vi "ReadAddErrorCase__slk_mt.vi"(8 "error in (no error)":errorcluster, 11 "refnum in":T1) -> (0 "error out":errorcluster, 2 "add error case configure":T2, 3 "refnum out":T1)   [LabVIEW 2020, in "Lazyboots Menu Tool.lvlib"]
doc: "Gets configure datum of Add Error Case.\n\n<b>[Add Error Case]</b>\nFrame Width = \"20\"\nCreate Constant = \"TRUE\""
uses:
  Library/Lazyboots Menu Tool.lvlib
  TypeDef/TypeDef_AddErrorCaseConfigure__slk_mt.ctl
  <vilib>/Utility/config.llb/Config Data RefNum.ctl
  <vilib>/Utility/config.llb/Read Key (U32).vi
  <vilib>/Utility/config.llb/Read Key (Boolean).vi
  <vilib>/Utility/config.llb/NI_LVConfig.lvlib
panel:
  # "ReadAddErrorCase__slk_mt.vi\nGets configure datum of Add Error Case.\n\nNOTICE -- YOU MUST LEAVE THIS NOTICE IN PLACE.\n\nCopyright (c) 2011, LIANG LIU Shawn.Liu.cn@gmail.com\nAll rights reserved.\n\nRedistribution and use in source and binary forms, with or without modification, are permitted provided that the following conditions are met:\n-Redistributions of source code must retain the above copyright notice, this list of conditions and the following disclaimer.\n-Redistributions in binary form must reproduce the above copyright notice, this list of conditions and the following disclaimer in the documentation and/or other materials provided with the distribution.\n-Neither the name of the eLp nor the names of its contributors may be used to endorse or promote products derived from this software without specific prior written permission.\n\nTHIS SOFTWARE IS PROVIDED BY THE COPYRIGHT HOLDERS AND CONTRIBUTORS \"AS IS\" AND ANY EXPRESS OR IMPLIED WARRANTIES, INCLUDING, BUT NOT LIMITED TO, THE IMPLIED WARRANTIES OF MERCHANTABILITY AND FITNESS FOR A PARTICULAR PURPOSE ARE DISCLAIMED. IN NO EVENT SHALL THE COPYRIGHT HOLDER OR CONTRIBUTORS BE LIABLE FOR ANY DIRECT, INDIRECT, INCIDENTAL, SPECIAL, EXEMPLARY, OR CONSEQUENTIAL DAMAGES (INCLUDING, BUT NOT LIMITED TO, PROCUREMENT OF SUBSTITUTE GOODS OR SERVICES; LOSS OF USE, DATA, OR PROFITS; OR BUSINESS INTERRUPTION) HOWEVER CAUSED AND ON ANY THEORY OF LIABILITY, WHETHER IN CONTRACT, STRICT LIABILITY, OR TORT (INCLUDING NEGLIGENCE OR OTHERWISE) ARISING IN ANY WAY OUT OF THE USE OF THIS SOFTWARE, EVEN IF ADVISED OF THE POSSIBILITY OF SUCH DAMAGE."
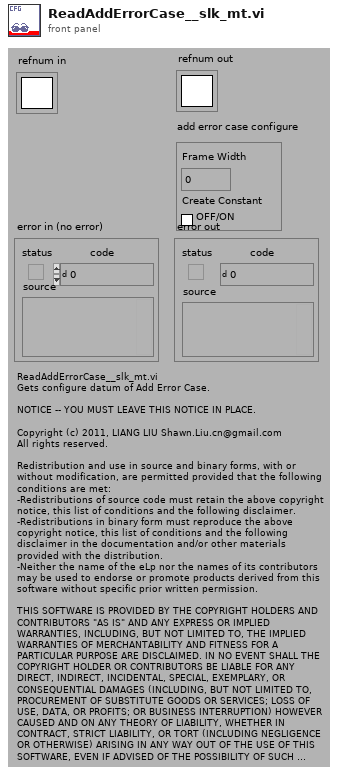
[diagram p1: front panel]
types:
  T1 = typedef "NI_LVConfig.lvlib/Config Data RefNum.ctl" = refnum<k1>
  T2 = typedef "Lazyboots Menu Tool.lvlib/TypeDef_AddErrorCaseConfigure__slk_mt.ctl" = cluster{"Frame Width":u32, "Create Constant":bool}
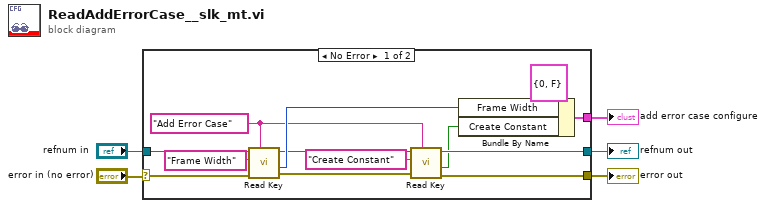
[diagram p0: block diagram]
diagram:
  n1 = case shown="No Error" "error in (no error)" {
    selector: "error in (no error)" -> [w15 w20]
    tunnel: "refnum in" -> [w18 w19]
    tunnel: [w9 w19] -> w4
    tunnel: [w14 _] -> w2
    tunnel: [w10 w20] -> w1
    frame No Error {
      w12 = "Add Error Case" ("section")
      n2 = call-poly <vilib>:"Read Key.vi"("section"=w12, "error in (no error)"=w15, "key"="Frame Width", "refnum"=w18) -> ("error out"=w11:errorcluster, "value"=w16:u32, "refnum out"=w8:T1)  [unwired: 4 in, 1 out]
      n3 = call-poly <vilib>:"Read Key.vi"("section"=w12, "error in (no error)"=w11, "key"="Create Constant", "refnum"=w8) -> ("error out"=w10:errorcluster, "value"=w7:bool, "refnum out"=w9:T1)  [unwired: 4 in, 1 out]
      n4 = Bundle By Name(cluster=T2 {"Frame Width"=0, "Create Constant"=FALSE} ("Add Error Casel Configure"), "Frame Width"=w16, "Create Constant"=w7) -> (w14:T2)
    }
    frame Error {
    }
  }
  "add error case configure" <- w2
  "error out" <- w1
  "refnum out" <- w4
